vi "SI SwitchVoltage.vi"(8 "error in (no error)":errorcluster, 10 "Boolean":bool, 11 "VISA Refnum in":refnum<visa-resource-name>) -> (0 "error out":errorcluster, 3 "Message":string)   [LabVIEW 2017]
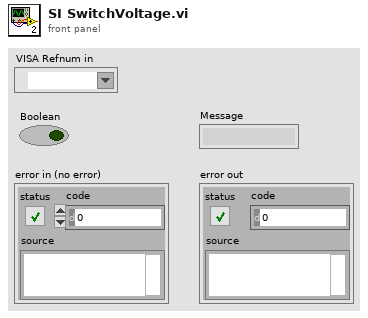
[diagram p1: front panel]
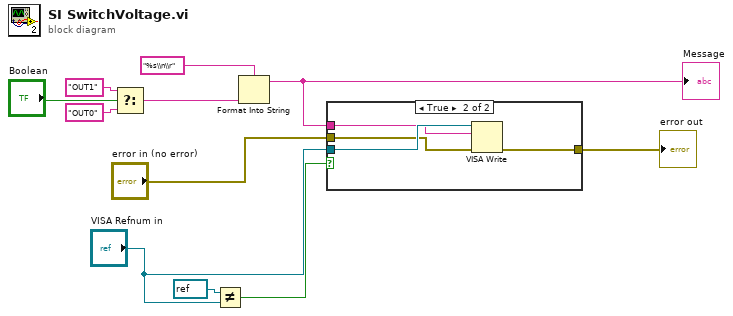
[diagram p0: block diagram]
diagram:
  n1 = Select(t="OUT1", s="Boolean", f="OUT0") -> (s? t:f=w8:string)
  n2 = Not Equal?(x=refnum<visa-resource-name> refnum ("Laser Port"), y="VISA Refnum in") -> (x != y?=w2:bool)
  n3 = Format Into String(format string="%s\\n\\r", w8) -> (resulting string=w9:string)  [unwired: 2 in, 1 out]
  "Message" <- w9
  n4 = case shown="True" w2 {
    tunnel: "VISA Refnum in" -> [_ w16]
    tunnel: "error in (no error)" -> [w12 w15]
    tunnel: [w12 w14] -> w11
    tunnel: w9 -> [_ w13]
    frame False {
    }
    frame True {
      n5 = VISA Write(VISA resource name=w16, write buffer=w13, error in (no error)=w15) -> (error out=w14:errorcluster)  [unwired: 2 out]
    }
  }
  "error out" <- w11
